vi "_Parse ACLR Segment Limit Check Result.vi"(8 "error in (no error)":errorcluster, 10 "Input String":string, 11 "VISA resource name":refnum<visa-resource-name>) -> (0 "error out":errorcluster, 1 "ACLR Results":T2, 2 "Reliability Results":T1, 3 "VISA resource name out":refnum<visa-resource-name>, 5 "Out Of Tolerance":dbl format="%^.3e", 7 "Statistic Expired":i32)   [LabVIEW 2020, in "Rohde&Schwarz CMXP NR FR2 Measurement.lvlib"]
uses:
  <instrlib>/Rohde&Schwarz CMXP NR FR2 Measurement/Rohde&Schwarz CMXP NR FR2 Measurement.lvlib
  <instrlib>/Rohde&Schwarz CMXP NR FR2 Measurement/Private/rsidr_core.llb/rsidr_core.lvlib
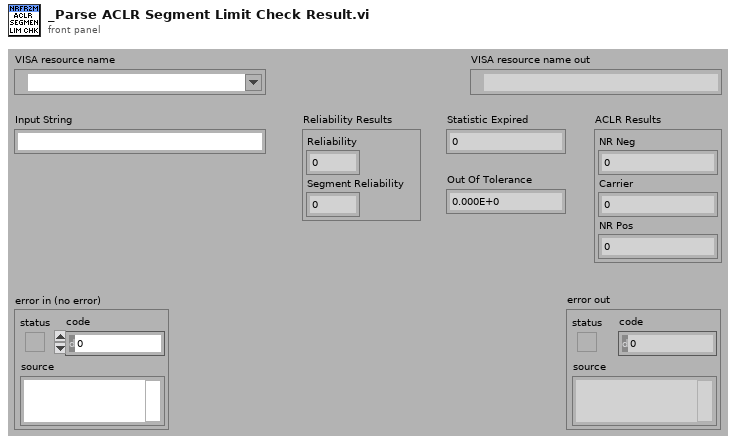
[diagram p1: front panel]
types:
  T1 = cluster{"Reliability":i32, "Segment Reliability":i32}
  T2 = cluster{"NR Neg":i32, "Carrier":i32, "NR Pos":i32}
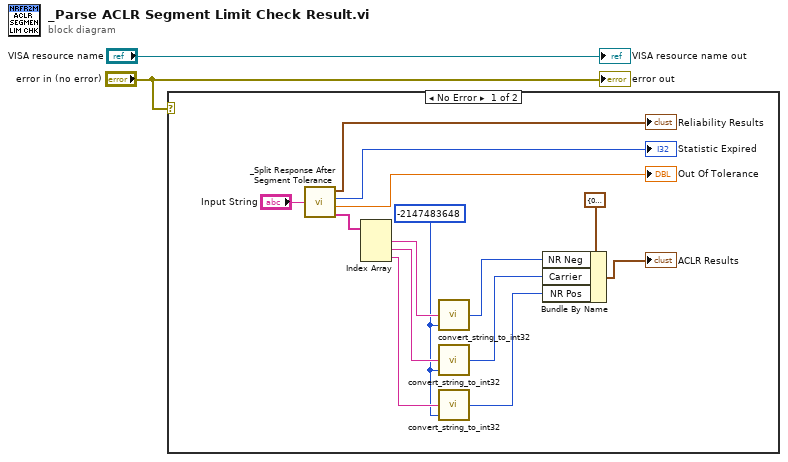
[diagram p0: block diagram]
diagram:
  n1 = case shown="No Error" "error in (no error)" {
    frame No Error {
      w7 = -2147483648
      n2 = call <instrlib>:"_Split Response After Segment Tolerance.vi"("Input String"="Input String") -> ("Reliability Results"=→"Reliability Results":T1, "Statistic Expired"=→"Statistic Expired":i32, "Out Of Tolerance"=→"Out Of Tolerance":dbl, "Response out"=w14:string[])
      n3 = Index Array(array=w14) -> (element #1=w13:string, element #2=w10:string, element #3=w11:string)  [unwired: 3 in]
      n4 = call <instrlib>:"convert_string_to_int32.vi"("default (0)"=w7, "String in"=w13) -> ("int32 value out"=w16:i32)  [unwired: 3 in]
      n5 = call <instrlib>:"convert_string_to_int32.vi"("default (0)"=w7, "String in"=w10) -> ("int32 value out"=w9:i32)  [unwired: 3 in]
      n6 = call <instrlib>:"convert_string_to_int32.vi"("default (0)"=w7, "String in"=w11) -> ("int32 value out"=w12:i32)  [unwired: 3 in]
      n7 = Bundle By Name(cluster=T2 {"NR Neg"=0, "Carrier"=0, "NR Pos"=0} ("ACLR Results"), "NR Neg"=w16, "Carrier"=w9, "NR Pos"=w12) -> (→"ACLR Results":T2)
    }
    frame Error {
    }
  }
  "error out" <- "error in (no error)"
  "VISA resource name out" <- "VISA resource name"
